vi "Set Sequence.vi"(8 "error in (no error)":errorcluster, 10 "Sequence":refnum<class "Sequence.lvclass">, 11 "Sequencer in":refnum<class "Sequencer.lvclass">) -> (0 "error out":errorcluster, 3 "Service out":refnum<class "Sequencer.lvclass">)   [LabVIEW 2024, in "Ramses Sequencer.lvlib" / "Sequencer.lvclass"]
uses:
  Sequencer.lvclass
  Sequence/Sequence.lvclass
  Program Files (x86)/Enterative/Ramses Framework/Ramses Framework.lvlibp/Service/Service.lvclass
  C:/Program Files (x86)/Enterative/Ramses Framework/Ramses Framework.lvlibp/Service/Service.lvclass
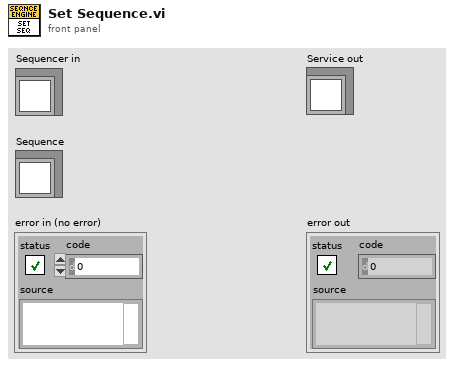
[diagram p1: front panel]
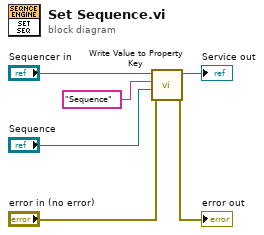
[diagram p0: block diagram]
diagram:
  n1 = call "Write Value to Property Key.vi"("error in (no error)"="error in (no error)", "Value"="Sequence", "Key"="Sequence", "Service in"="Sequencer in") -> ("error out"=→"error out":errorcluster, "Service out"=→"Service out":refnum<class "Sequencer.lvclass">)  [unwired: 6 in]
